vi "Voltage Min Read Single.vi"(8 "error in":errorcluster, 9 "Channel Index":i32=1, 11 "Cycler in":refnum<class "Cycler.lvclass">) -> (0 "error out":errorcluster, 1 "Changed or First Call?":bool, 2 "Voltage Min SP":dbl, 3 "Cycler out":refnum<class "Cycler.lvclass">)   [LabVIEW 2023, in "Cycler.lvclass"]
uses:
  Cycler.lvclass
  Cycler.lvclass/Cycler.ctl
  Low Level Capabilities/Voltage/Voltage Limit/Voltage Limit.lvclass
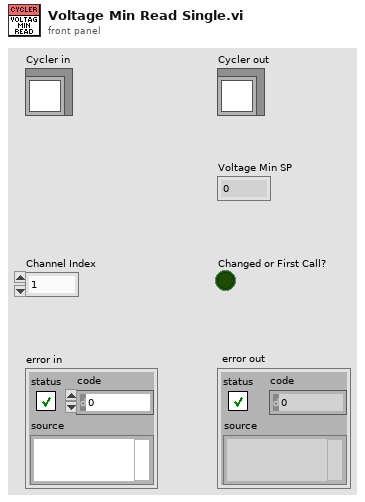
[diagram p1: front panel]
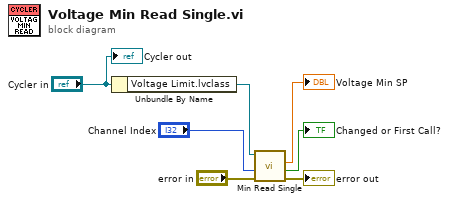
[diagram p0: block diagram]
diagram:
  n1 = Unbundle By Name("Cycler in") -> ("Voltage Limit.lvclass"=w7:refnum<class "Voltage Limit.lvclass">)
  n2 = call-dynamic "Min Read Single.vi"("error in"="error in", "Channel Index"="Channel Index", "Min Voltage Limit in"=w7) -> ("error out"=→"error out":errorcluster, "Changed or First Call?"=→"Changed or First Call?":bool, "Voltage Min SP"=→"Voltage Min SP":dbl)  [unwired: 5 in, 1 out]
  "Cycler out" <- "Cycler in"
